vi "Configure RF Resolution Bandwidth.vi"(0 "VISA resource name":refnum<visa-resource-name>, 1 "Auto Resolution (T: Enable)":bool=TRUE, 2 "Auto Reference Level (T: Enable)":bool=TRUE, 5 "RF Window Function (0:Kaiser)":u16(ring) items=["Kaiser", "Rectangular", "Hamming", "Hanning", "Blackman-Harris", "Flat-Top"], 7 "Span: Bandwidth Ratio (1000:1)":dbl=1000.0 format="%#_g : 1", 9 "Manual Resolution (55 Hz)":dbl=55.0, 11 "error in (no error)":errorcluster, 12 "Units (0: Hz)":u16(ring) items=["Hz", "kHz"], 13 "Manual Reference (30 dBm)":dbl=30.0, 14 "Units (0: dBm)":u16(ring) items=["dBm", "dBµW", "dBmV", "dbµV", "dbmA", "dBµA"]) -> (4 "VISA resource name out":refnum<visa-resource-name>, 15 "error out":errorcluster)   [LabVIEW 2009, in "Tektronix DPO MSO 2000 4000 Series.lvlib"]
doc: "Configures the Window function, Span:Bandwidth Ratio, Reference Level and Resolution Bandwidth for MDO Series Oscilloscopes.\n\n<B>Note:</B>\n This VI is only applicable to <B>MDO series</B> oscilloscopes."
uses:
  <instrlib>/Tektronix DPO MSO 2000 4000 Series/Tektronix DPO MSO 2000 4000 Series.lvlib
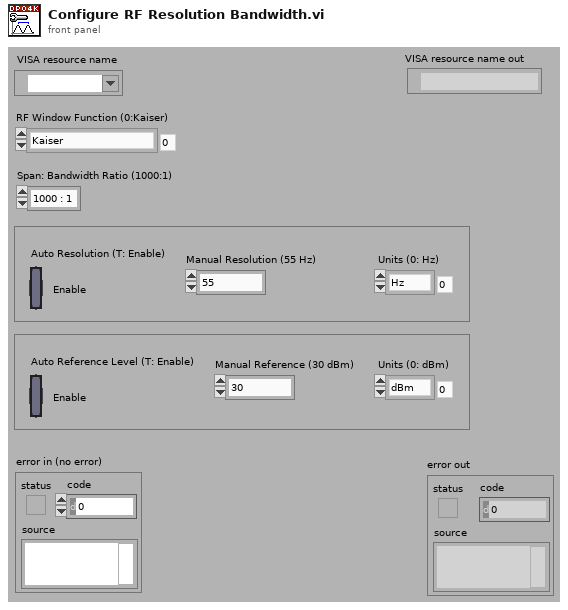
[diagram p1: front panel]
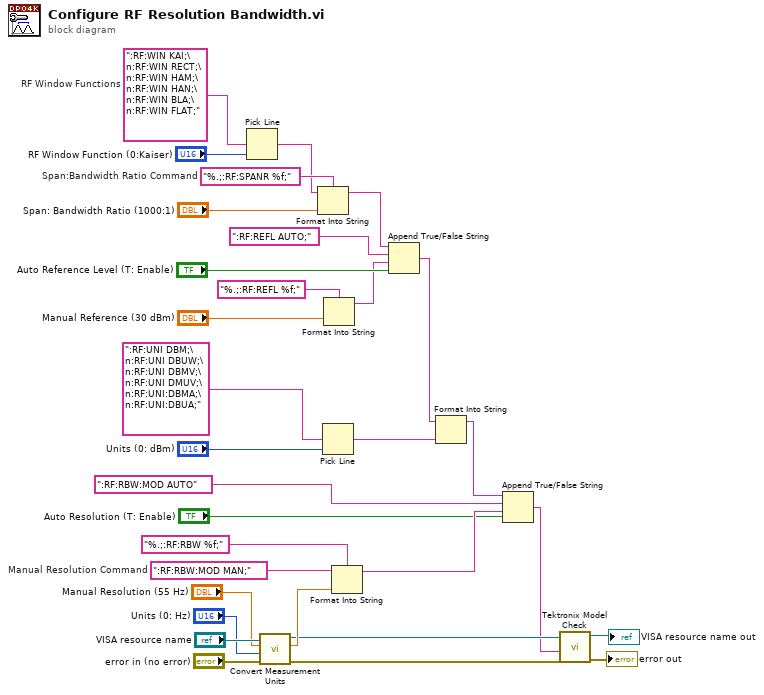
[diagram p0: block diagram]
diagram:
  w9 = ":RF:RBW:MOD MAN;"  # Manual Resolution Command
  w29 = "%.;:RF:SPANR %f;"  # Span:Bandwidth Ratio Command
  w30 = ":RF:WIN KAI;\n:RF:WIN RECT;\n:RF:WIN HAM;\n:RF:WIN HAN;\n:RF:WIN BLA;\n:RF:WIN FLAT;"  # RF Window Functions
  n1 = Pick Line(multi-line string=w30, line index="RF Window Function (0:Kaiser)") -> (output string=w27:string)  [unwired: 1 in]
  n2 = call <instrlib>:"Convert Measurement Units.vi"("error in (no error)"="error in (no error)", "Units (0:Hz)"="Units (0: Hz)", "Measurement Value (0)"="Manual Resolution (55 Hz)", "VISA resource name"="VISA resource name") -> ("error out"=w3:errorcluster, "Final Value"=w11:dbl, "VISA resource name out"=w5:refnum<visa-resource-name>)  [unwired: 5 in]
  n3 = Format Into String(format string=w29, initial string=w27, "Span: Bandwidth Ratio (1000:1)") -> (resulting string=w24:string)  [unwired: 1 in, 1 out]
  n4 = Pick Line(multi-line string=":RF:UNI DBM;\n:RF:UNI DBUW;\n:RF:UNI DBMV;\n:RF:UNI DMUV;\n:RF:UNI:DBMA;\n:RF:UNI:DBUA;", line index="Units (0: dBm)") -> (output string=w17:string)  [unwired: 1 in]
  n5 = Format Into String(format string="%.;:RF:REFL %f;", "Manual Reference (30 dBm)") -> (resulting string=w21:string)  [unwired: 2 in, 1 out]
  n6 = Format Into String(format string="%.;:RF:RBW %f;", initial string=w9, w11) -> (resulting string=w8:string)  [unwired: 1 in, 1 out]
  n7 = Append True/False String(1:"Auto Reference Level (T: Enable)", 2:w21, 3:":RF:REFL AUTO;" ("true string"), 4:w24) -> (0:w20:string)
  n8 = Format Into String(initial string=w20, w17) -> (resulting string=w16:string)  [unwired: 2 in, 1 out]
  n9 = Append True/False String(1:"Auto Resolution (T: Enable)", 2:w8, 3:":RF:RBW:MOD AUTO" ("true string"), 4:w16) -> (0:w4:string)
  n10 = call <instrlib>:"Tektronix Model Check.vi"("error in (no error)"=w3, "Command String"=w4, "VISA resource name"=w5) -> ("error out"=→"error out":errorcluster, "VISA resource name out"=→"VISA resource name out":refnum<visa-resource-name>)  [unwired: 7 in]
